vi "Write Config Changes to File.vi"(8 "error in (no error)":errorcluster, 10 "New Config":string="{}", 11 "Config File in":refnum<class "Config File.lvclass">) -> (0 "error out":errorcluster, 2 "<JSON>Config as Written":string, 3 "Config File":refnum<class "Config File.lvclass">, 4 "<JSON>As in file (before changes)":string)   [LabVIEW 2020, in "Config File.lvclass"]
doc: "Write changed configuration info to the Config File. Changes are defined as differences between the input \"New Config\" and the \"Original Config\" originally Read from the file. These changes are then applied to the current Config File. \n\nNot that non-conflicting changes made to the file by another application between \"Read Config\" and \"Write Config Changes\" will not be overwritten, as only items changed by this application will be altered. This allows multiple applications or code compoenents to maintain different parameters in the same config file, without issues of race condition overwrite (as long as different apps do not alter the same item)."
uses:
  <vilib>/JDP Science/JSONtext/Config Files/Config File.lvclass
  <vilib>/JDP Science/JSONtext/Config Files/Config File.lvclass/Config File.ctl
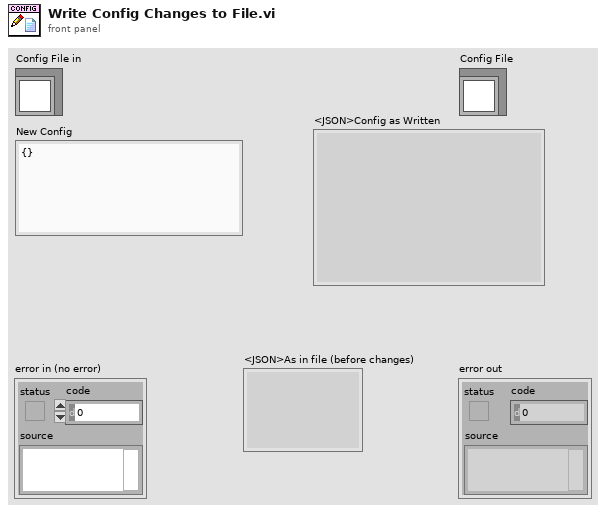
[diagram p1: front panel]
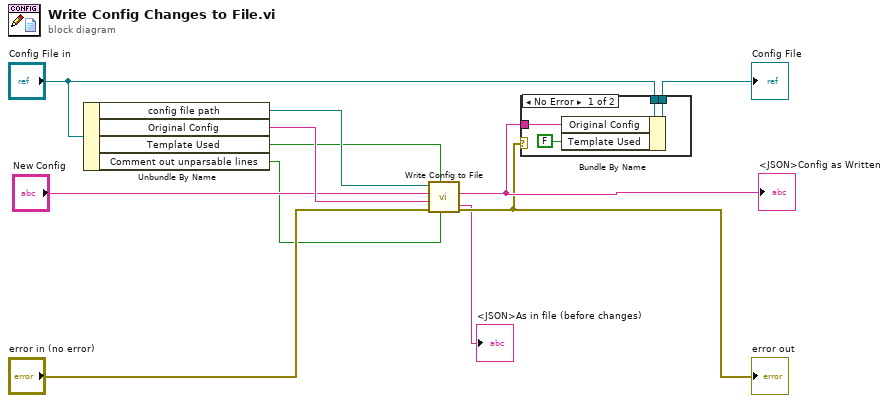
[diagram p0: block diagram]
diagram:
  n1 = Unbundle By Name("Config File in") -> ("config file path"=w8:path, "Original Config"=w9:string, "Template Used"=w6:bool, "Comment out unparsable lines"=w2:bool)
  n2 = call <vilib>:"Write Config to File.vi"("Comment out unparsable lines"=w2, "Write even if no changes"=w6, "error in (no error)"="error in (no error)", "Original Config"=w9, "New Config"="New Config", "config file path"=w8) -> ("error out"=w3:errorcluster, "<JSON>Config as Written"=w4:string, "<JSON>As in file (before changes)"=→"<JSON>As in file (before changes)":string)  [unwired: 3 in]
  "error out" <- w3
  "<JSON>Config as Written" <- w4
  n3 = case shown="No Error" w3 {
    tunnel: "Config File in" -> [w15 w16]
    tunnel: [w14 w16] -> w5
    tunnel: w4 -> [w13 _]
    frame No Error {
      n4 = Bundle By Name(cluster=w15, "Original Config"=w13, "Template Used"=FALSE) -> (w14:refnum<class "Config File.lvclass">)
    }
    frame Error {
    }
  }
  "Config File" <- w5
